vi "Call VI by Name.vi"(6 "Auto Dispose Ref":bool, 7 "FrontPanel(close)":T2(ring)=enum."Closed", 8 "error in":errorcluster, 9 "CtrlValue":variant, 10 "CtrlName":string, 11 "VI Name":string) -> (0 "错误输出":errorcluster caption="error out", 2 "Exec.State":T1(ring), 3 "Dynamic vi reference out":refnum<vi>)   [LabVIEW 2016, in "PanelRootNode.lvclass"]
uses:
  PanelRootNode.lvclass
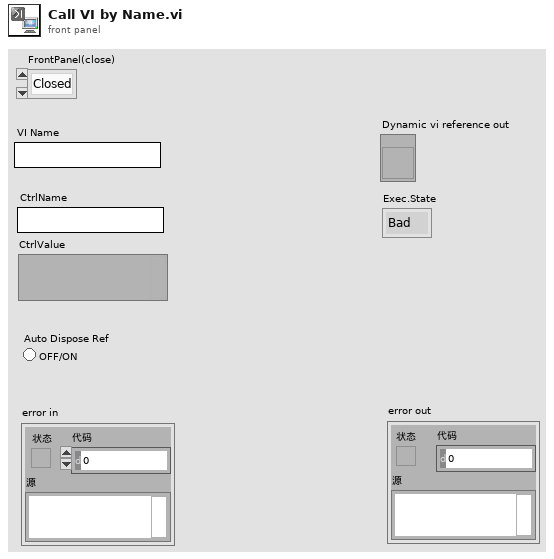
[diagram p1: front panel]
types:
  T1 = enum32{"Bad", "Idle", "Run top level", "Running"}
  T2 = enum32{"Invalid", "Standard", "Closed", "Hidden", "Minimized", "Maximized"}
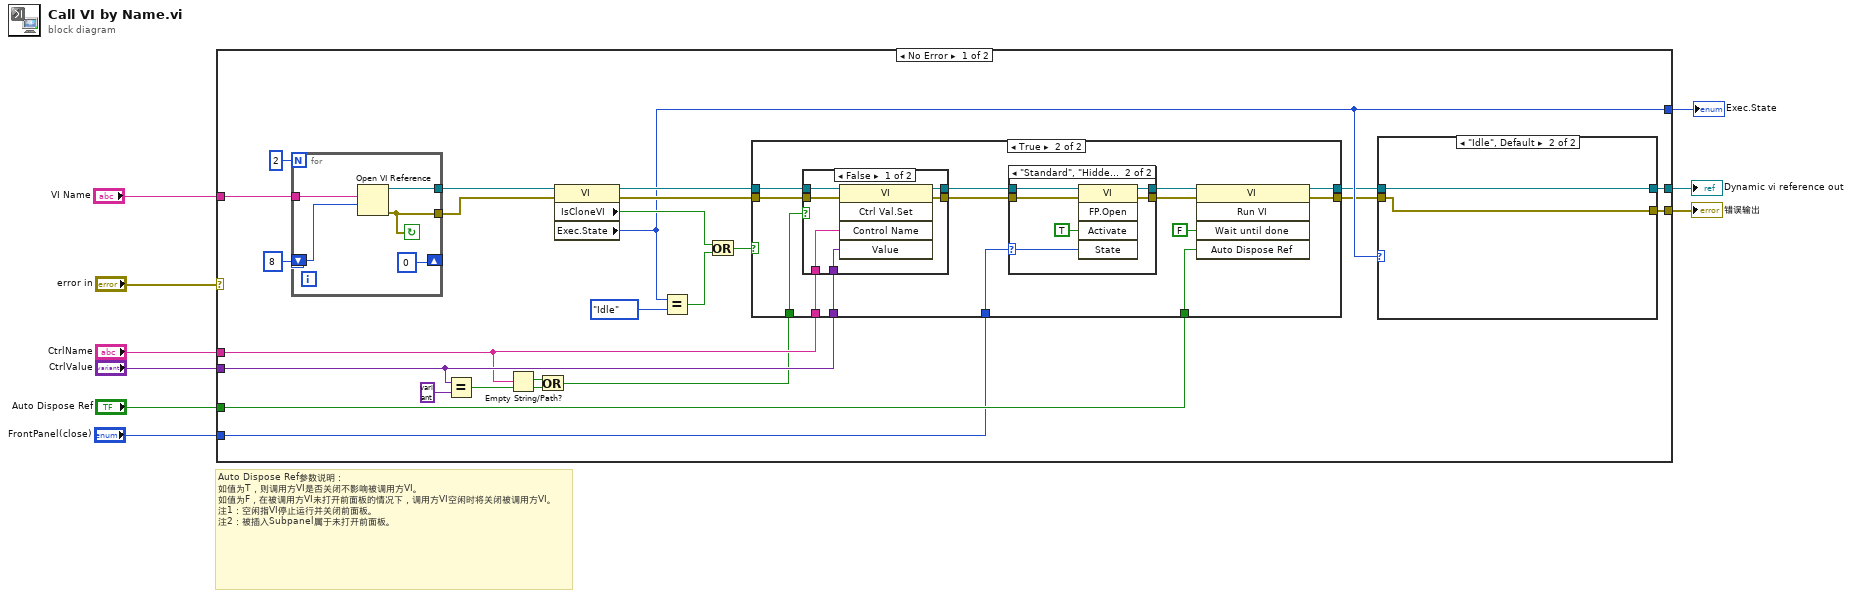
[diagram p0: block diagram]
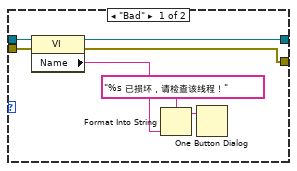
[diagram p2: hidden frame]
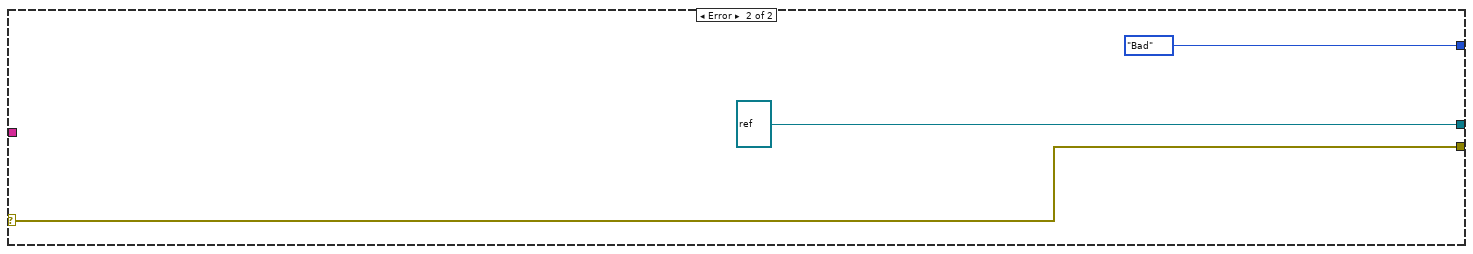
[diagram p6: hidden frame]
diagram:
  # "Auto Dispose Ref参数说明：\n如值为T，则调用方VI是否关闭不影响被调用方VI。\n如值为F，在被调用方VI未打开前面板的情况下，调用方VI空闲时将关闭被调用方VI。\n注1：空闲指VI停止运行并关闭前面板。\n注2：被插入Subpanel属于未打开前面板。"
  n1 = case shown="No Error" "error in" {
    selector: "error in" -> [_ w81]
    tunnel: [w11 refnum<vi> refnum ("vi reference")] -> w9
    tunnel: [w10 w81] -> w8
    tunnel: "Auto Dispose Ref" -> [w25 _]
    tunnel: "CtrlName" -> [w22 _]
    tunnel: "CtrlValue" -> [w24 _]
    tunnel: "VI Name" -> [w18 _]
    tunnel: "FrontPanel(close)" -> [w17 _]
    tunnel: [w14 T1."Bad" ("Exec.State")] -> w3
    frame No Error {
      n2 = for {
        N: 2 -> [_]
        tunnel: w18 -> [w47]
        shift-right: [0 ("选项")] -> _
        shift-left: 8 ("选项") -> [w46]
        tunnel: [w44] -> w15
        tunnel: [w43] -> w16
        stop <- w44 continue-if-true
        n3 = Open VI Reference(vi path=w47, options=w46) -> (vi reference=w43:refnum<vi>, error out=w44:errorcluster)  [unwired: 4 in]
      }
      n4 = Equal?(x=w24, y=variant) -> (x = y?=w20:bool)
      n5 = Empty String/Path?(string/path=w22) -> (empty?=w21:bool)
      n6 = Or(x=w21, y=w20) -> (x .or. y?=w19:bool)
      n7 = property class="VI"(reference=w16, error in=w15) -> (reference out=w33:refnum<vi>, error out=w32:errorcluster, "IsCloneVI"=w28:bool, "Exec.State"=w14:T1)
      n8 = Equal?(x=w14, y=T1."Idle") -> (x = y?=w27:bool)
      n9 = Or(x=w28, y=w27) -> (x .or. y?=w26:bool)
      n10 = case shown="True" w26 {
        tunnel: w33 -> [w49 w59]
        tunnel: [w49 w63] -> w13
        tunnel: w32 -> [w48 w58]
        tunnel: [w48 w62] -> w12
        tunnel: w25 -> [_ w60]
        tunnel: w22 -> [_ w57]
        tunnel: w24 -> [_ w56]
        tunnel: w19 -> [_ w55]
        tunnel: w17 -> [_ w50]
        frame False {
        }
        frame True {
          n11 = case shown="False" w55 {
            tunnel: w59 -> [w77 w79]
            tunnel: [w76 w79] -> w54
            tunnel: w58 -> [w75 w78]
            tunnel: [w74 w78] -> w53
            tunnel: w57 -> [w73 _]
            tunnel: w56 -> [w72 _]
            frame False {
              n12 = invoke class="VI" method="Ctrl Val.Set"(reference=w77, error in=w75, "Control Name"=w73, "Value"=w72) -> (reference out=w76:refnum<vi>, error out=w74:errorcluster)  [unwired: 1 in, 3 out]
            }
            frame True {
            }
          }
          n13 = case shown="\"Standard\", \"Hidden\"..\"Maximized\"" w50 {
            selector: w50 -> [_ w66]
            tunnel: w54 -> [w65 w71]
            tunnel: w53 -> [w64 w70]
            tunnel: [w65 w69] -> w52
            tunnel: [w64 w68] -> w51
            frame "Invalid", Default {
            }
            frame "Standard", "Hidden".."Maximized" {
              n14 = invoke class="VI" method="FP.Open"(reference=w71, error in=w70, "Activate"=TRUE ("激活？"), "State"=w66) -> (reference out=w69:refnum<vi>, error out=w68:errorcluster)  [unwired: 1 in, 3 out]
            }
          }
          n15 = invoke class="VI" method="Run VI"(reference=w52, error in=w51, "Wait until done"=FALSE ("结束前等待"), "Auto Dispose Ref"=w60) -> (reference out=w63:refnum<vi>, error out=w62:errorcluster)  [unwired: 1 in, 3 out]
        }
      }
      n16 = case shown="\"Idle\", Default" w14 {
        tunnel: w13 -> [w37 w42]
        tunnel: w12 -> [w38 w41]
        tunnel: [w35 w42] -> w11
        tunnel: [w34 w41] -> w10
        frame "Bad" {
          n17 = property class="VI"(reference=w37, error in=w38) -> (reference out=w35:refnum<vi>, error out=w34:errorcluster, "Name"=w36:string)
          n18 = Format Into String(format string="%s 已损坏，请检查该线程！" ("格式字符串"), w36) -> (resulting string=w40:string)  [unwired: 2 in, 1 out]
          n19 = One Button Dialog(message=w40) -> ()  [unwired: 1 in, 1 out]
        }
        frame "Idle", Default {
        }
      }
    }
    frame Error {
    }
  }
  "Dynamic vi reference out" <- w9
  "错误输出" <- w8
  "Exec.State" <- w3
